vi "FTW-JSON-RegexParse.vi"(0 "Regular Expression using JSON subroutines":string, 5 "Input String":string, 9 "Starting Offset":i32, 11 "error in":errorcluster) -> (4 "Match":string, 6 "Submatches":string[](array[string]), 8 "Found Match?":bool, 10 "Offset after Match":i32, 15 "error out":errorcluster)   [LabVIEW 2013]
panel:
  # "Inputs"
  # "Outputs"
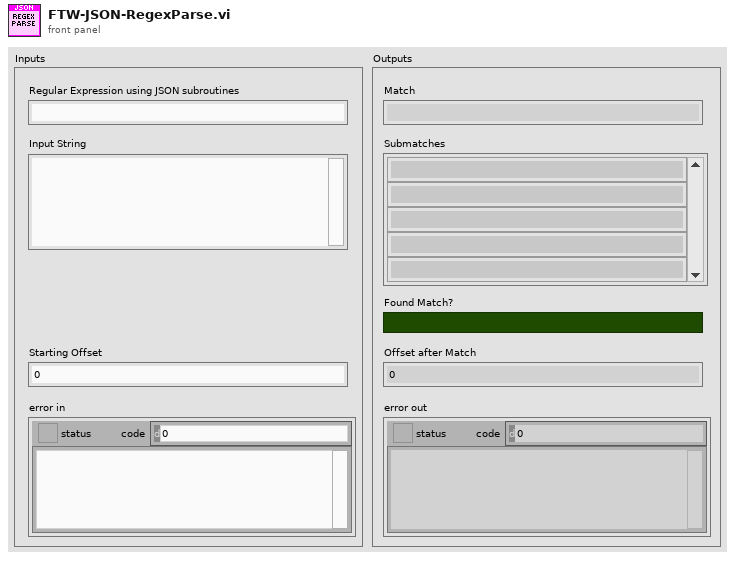
[diagram p1: front panel]
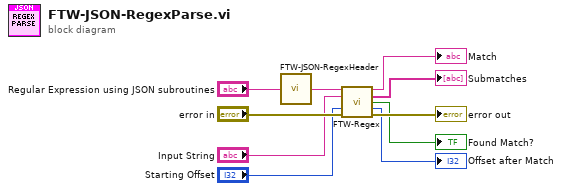
[diagram p0: block diagram]
diagram:
  n1 = call "FTW-JSON-RegexHeader.vi"("Regular Expression Body"="Regular Expression using JSON subroutines") -> ("Regular Expression with Header"=w6:string)
  n2 = call "FTW-Regex.vi"("Regular Expression"=w6, "Input String"="Input String", "Starting Offset"="Starting Offset", "error in"="error in") -> ("Match"=→"Match":string, "Submatches"=→"Submatches":string[], "Match Found?"=→"Found Match?":bool, "Offset after Match"=→"Offset after Match":i32, "error out"=→"error out":errorcluster)  [unwired: 7 in]
